vi "LIA Lock-In Simulation.vi"() -> ()   [LabVIEW 2017]
uses:
  <vilib>/Analysis/4window.llb/windowTd.ctl
  <vilib>/measure/maspectr.llb/FFT Power Spectrum and PSD for 1 Chan (CDB).vi
  <instrlib>/niRFSG/niRFSG.llb/niRFSG Fractional Resampling (I-Q).vi
  <vilib>/addons/Digital Filter Design/Multirate.llb/DFD MRate Filtering (Array).vi
  <vilib>/measure/maspectr.llb/FFT Power Spectrum and PSD for 1 Chan.vi
  <vilib>/addons/Digital Filter Design/NI_DigFilterLicensed.lvlib
  <vilib>/ptbypt/NI_PtbyPt.lvlib
  <vilib>/measure/NI_MAPro.lvlib
  <vilib>/Analysis/NI_AALPro.lvlib
panel:
  out "r max - min":dbl=0.5000000090754294 format="%#_6p"
  out "r min":dbl=0.5000000090754294 format="%#_6p"
  out "r max":dbl=0.5000000090754294 format="%#_6p"
  out "Waveform Graph 4":dbl[][](graph) caption="Filtered Response - Time"
  out "r mean":dbl=0.5000000090754294 format="%#_6p"
  in  "sample length":i32=4096
  in  "frequency error (Hz)":dbl format="%#_6p"
  out "Waveform Graph 3":cluster{"f0":dbl, "df":dbl, "magnitude":dbl[]}(graph) caption="Filtered Response - Frequency"
  out "Waveform Graph 2":cluster{"f0":dbl, "df":dbl, "magnitude":dbl[]}[](graph)
  in  "noise":dbl=0.0001 format="%.2p"
  in  "fs":dbl=100000000.0 format="%#_6p"
  in  "decimating factor":i32=1000
  out "error out":errorcluster
  in  "signal freq":dbl=100000.0 format="%#_6p"
  in  "stop":bool
  out "filter response":cluster{"f0":dbl, "df":dbl, "values":dbl[]}[](graph)
  out "Waveform Graph":dbl[][](graph) caption="Filtered Response - Time"
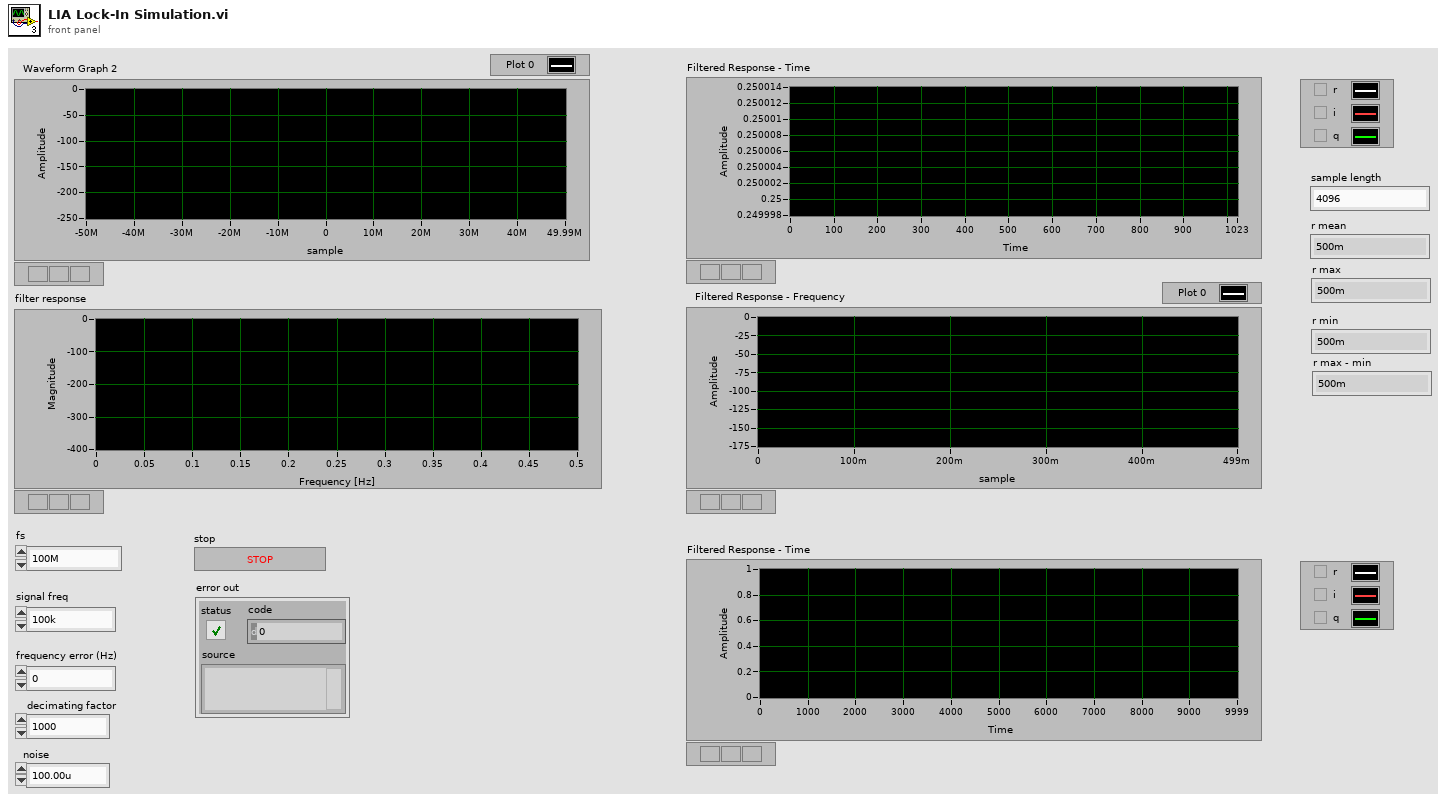
[diagram p1: front panel]
types:
  T1 = typedef "NI_AALPro.lvlib/windowTd.ctl" = u32
  T2 = typedef "NI_DigFilterLicensed.lvlib/DFD Multirate Filter Obj.ctl" = cluster{"mMRate_Structure":enum16{"CIC", "FIR", "IIR", "Lattice"}, "mMRate_Mode":T3, "mMRate_Factor":i32, "mMRate_FIRParams":cluster{"mMRate_FIR_H":dbl[], "mMRate_FIR_IsNyquist?":bool, "mMRate_FIR_IsSymmetric?":bool}, "mMRate_CICParams":cluster{"mMRate_CIC_#Stage":i32, "mMRate_CIC_Lag":i32, "mMRate_CIC_Type":enum16{"Lowpass", "Highpass"}}, "mMRate_Order":i32, "mMRate_Version":string, "mMRate_Comments":string, "mMRate_RationalFactor":cluster{"mMRate_L":i32, "mMRate_M":i32}, "mMRate_Fs":dbl, "mMRate_Quantized?":bool, "mMRate_QFilterGain":dbl, "mMRate_CoefWl":i16, "mMRate_Scaling":cluster{"mMRate_ScaleByPowerOf2?":bool, "mMRate_ScaleType":T4}, "mMRate_InputWl":i16, "mMRate_OutputWl":i16, "mMRate_OutputMode":T5, "mMRate_MultMode":T6, "mMRate_BitPruning":bool, "mMRate_GainWl":i16, "mMRate_OutputFwl":i16, "mMRate_SumIwl":i16, "mMRate_InputIwl ":i16, "mMRate_SumWl":i16, "mMRate_CoefIwl":i16}
  T3 = typedef "NI_DigFilterLicensed.lvlib/DFD Multirate Mode.ctl" = i16
  T4 = typedef "NI_DigFilterLicensed.lvlib/DFD Coef Norm Type.ctl" = enum16{"No Norm", "Time Domain 1-Norm", "Time Domain 2-Norm", "Time Domain Inf-Norm"}
  T5 = typedef "NI_DigFilterLicensed.lvlib/DFD Round-off Mode.ctl" = enum16{"Nearest", "Truncation"}
  T6 = typedef "NI_DigFilterLicensed.lvlib/DFD FXP MRate Multiply Mode.ctl" = enum16{"Truncated", "Full"}
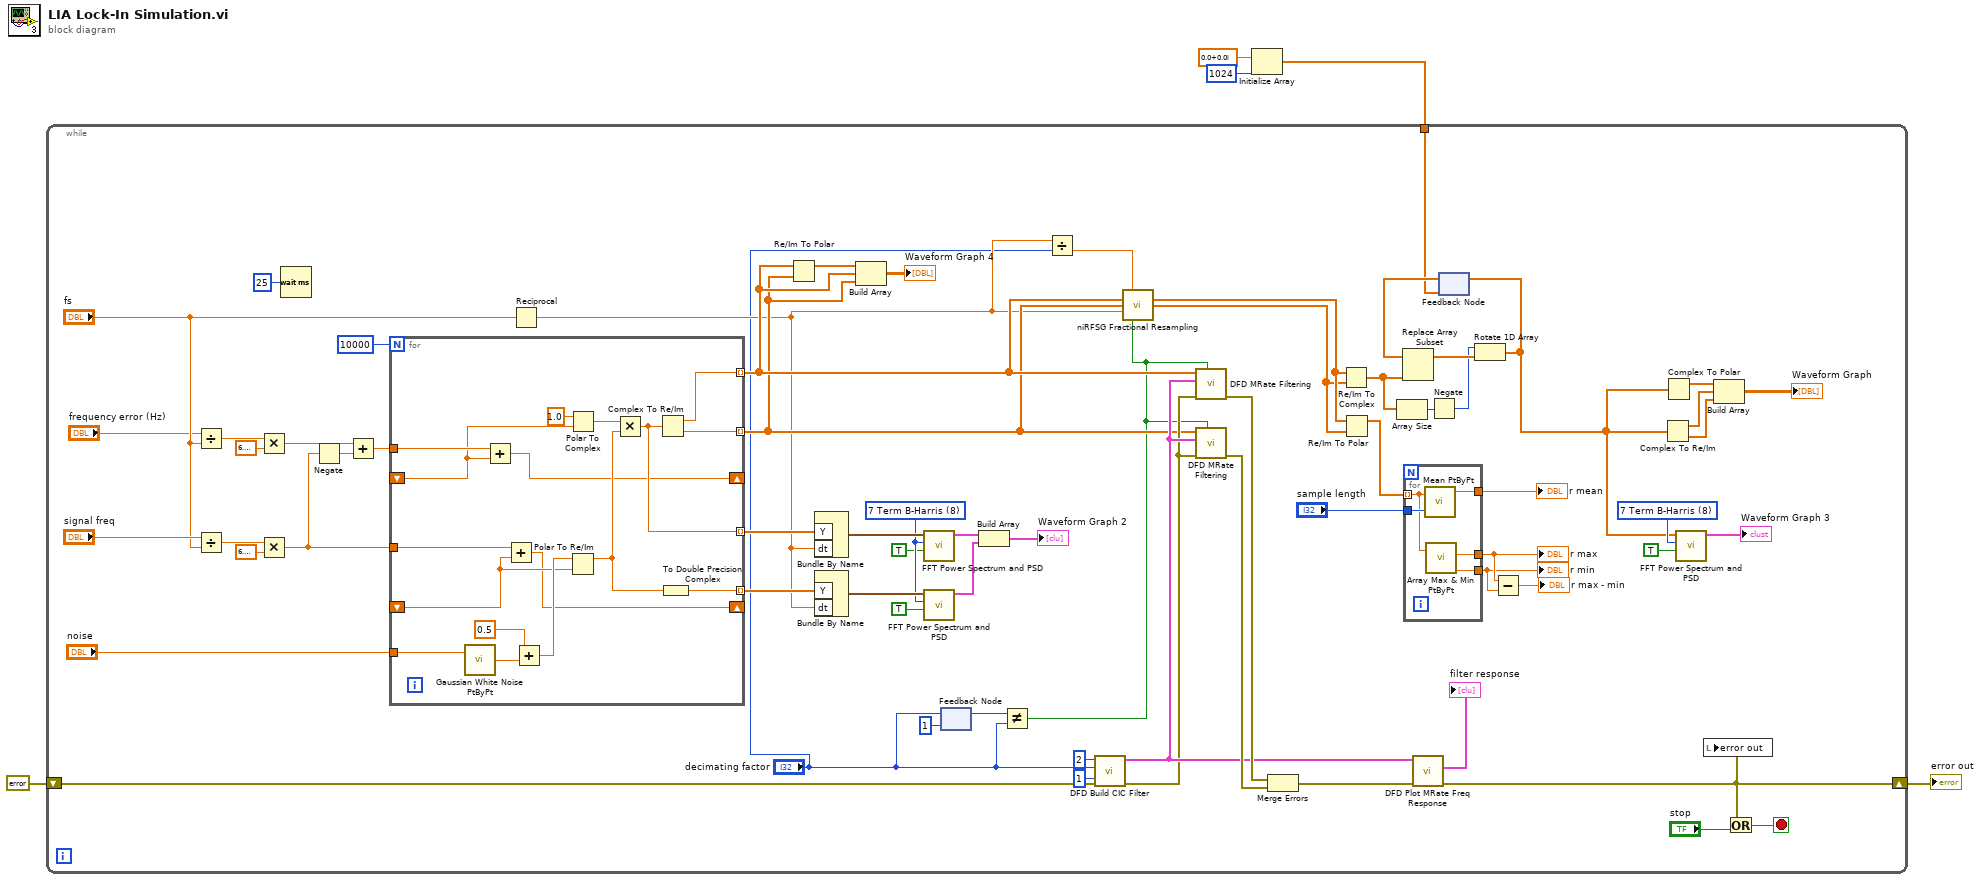
[diagram p0: block diagram]
diagram:
  n1 = Initialize Array(cdb 0.0+0.0i ("element"), 1024 ("dimension size")) -> (w1:cdb[])
  n2 = while {
    shift-right: [w60] -> w5
    shift-left: errorcluster {"status"=FALSE, "code"=0, "source"=""} ("error out") -> [w62]
    tunnel: w1 -> [w26]
    stop <- w67 stop-if-true
    w45 = T1 8 items=["Rectangle"=0, "Hanning"=1, "Hamming"=2, "Blackman-Harris"=3, "Exact Blackman"=4, "Blackman"=5, "Flat Top"=6, "4 Term B-Harris "=7, "7 Term B-Harris"=8, "Low Sidelobe"=9, "Blackman Nuttall"=11, "Triangle"=30, "Bartlett-Hanning"=31, "Bohman"=32, "Parzen"=33, "Welch"=34, "Kaiser"=60, "Dolph-Chebyshev"=61, "Gaussian"=62] ("window")
    w52 = T1 8 items=["Rectangle"=0, "Hanning"=1, "Hamming"=2, "Blackman-Harris"=3, "Exact Blackman"=4, "Blackman"=5, "Flat Top"=6, "4 Term B-Harris "=7, "7 Term B-Harris"=8, "Low Sidelobe"=9, "Blackman Nuttall"=11, "Triangle"=30, "Bartlett-Hanning"=31, "Bohman"=32, "Parzen"=33, "Welch"=34, "Kaiser"=60, "Dolph-Chebyshev"=61, "Gaussian"=62] ("window")
    n3 = Divide(x="frequency error (Hz)", y="fs") -> (x/y=w34:dbl)
    n4 = Divide(x="signal freq", y="fs") -> (x/y=w59:dbl)
    n5 = Multiply(x=w34, y=6.283185307179586) -> (x*y=w30:dbl)
    n6 = Multiply(x=w59, y=6.283185307179586) -> (x*y=w37:dbl)
    n7 = Wait (ms)(milliseconds to wait=u32 25) -> ()  [unwired: 1 out]
    n8 = Negate(x=w37) -> (-x=w41:dbl)
    n9 = Add(x=w30, y=w41) -> (x+y=w36:dbl)
    n10 = for {
      N: 10000 -> [_]
      tunnel: w36 -> [w83]
      tunnel: [w93] -> w13 mode=indexing
      tunnel: [w92] -> w12 mode=indexing
      tunnel: w37 -> [w82]
      tunnel: "noise" -> [w88]
      tunnel: [w85] -> w55 mode=indexing
      tunnel: [w86] -> w56 mode=indexing
      shift-right: [w84] -> _
      shift-left: _ -> [w79]
      shift-right: [w80] -> _
      shift-left: _ -> [w81]
      n11 = call <vilib>:"Gaussian White Noise PtByPt.vi"("standard deviation"=w88) -> ("Gaussian white noise"=w91:dbl)  [unwired: 2 in]
      n12 = Add(x=w83, y=w79) -> (x+y=w84:dbl)
      n13 = Add(x=w82, y=w81) -> (x+y=w80:dbl)
      n14 = Add(x=0.5 ("r"), y=w91) -> (x+y=w89:dbl)
      n15 = Polar To Complex(1:w79, 2:1.0 ("r")) -> (0:w94:cdb)
      n16 = Polar To Re/Im(2:w81, 3:w89) -> (1:w87:dbl)  [unwired: 1 out]
      n17 = Multiply(x=w94, y=w87) -> (x*y=w86:cdb)
      n18 = Complex To Re/Im(x + iy=w86) -> (x=w93:dbl, y=w92:dbl)
      n19 = To Double Precision Complex(1:w87) -> (0:w85:cdb)
    }
    n20 = Reciprocal(x="fs") -> (1/x=w11:dbl)
    n21 = Re/Im To Polar(2:w12, 3:w13) -> (1:w19:dbl[])  [unwired: 1 out]
    n22 = Bundle By Name("Y"=w56, "dt"=w11) -> (w54:waveform(cdb))  [unwired: 1 in]
    n23 = Bundle By Name("Y"=w55, "dt"=w11) -> (w53:waveform(cdb))  [unwired: 1 in]
    n24 = Build Array(w19, w13, w12) -> (→"Waveform Graph 4":dbl[][])
    n25 = call-poly <vilib>:"FFT Power Spectrum and PSD.vi"("dB On (F)"=TRUE, "window"=w52, "time signal"=w54) -> ("Power Spectrum / PSD"=w49:cluster{"f0":dbl, "df":dbl, "magnitude":dbl[]})  [unwired: 5 in, 3 out]
    n26 = call-poly <vilib>:"FFT Power Spectrum and PSD.vi"("dB On (F)"=TRUE, "window"=w52, "time signal"=w53) -> ("Power Spectrum / PSD"=w48:cluster{"f0":dbl, "df":dbl, "magnitude":dbl[]})  [unwired: 5 in, 3 out]
    n27 = feedback-in #1("decimating factor") -> ()
    n28 = feedback #1(1 ("decimating factor")) -> (w43:i32)
    n29 = Build Array(w49, w48) -> (→"Waveform Graph 2":cluster{"f0":dbl, "df":dbl, "magnitude":dbl[]}[])
    n30 = Not Equal?(x=w43, y="decimating factor") -> (x != y?=w8:bool)
    n31 = Divide(x=w11, y="decimating factor") -> (x/y=w10:dbl)
    n32 = call <vilib>:"DFD Build CIC Filter.vi"("error in (no error)"=w62, "differential delay"=1, "factor"="decimating factor", "# stages"=2) -> ("error out"=w61:errorcluster, "CIC filter out"=w63:T2)  [unwired: 6 in]
    n33 = call-poly <instrlib>:"niRFSG Fractional Resampling.vi"("desired sample rate (Hz)"=w10, "I"=w13, "Q"=w12, "input sample rate"=w11, "reset? (T)"=w8) -> ("I out"=w7:dbl[], "Q out"=w6:dbl[])  [unwired: 8 in, 1 out]
    n34 = call-poly <vilib>:"DFD MRate Filtering.vi"("init? (F)"=w8, "error in (no error)"=w61, "multirate filter"=w63, "signal in"=w13) -> ("error out"=w65:errorcluster)  [unwired: 6 in, 1 out]
    n35 = call-poly <vilib>:"DFD MRate Filtering.vi"("init? (F)"=w8, "error in (no error)"=w61, "multirate filter"=w63, "signal in"=w12) -> ("error out"=w68:errorcluster)  [unwired: 6 in, 1 out]
    n36 = Merge Errors(w65, w68) -> (w66:errorcluster)
    n37 = Re/Im To Complex(1:w6, 2:w7) -> (0:w28:cdb[])
    n38 = Re/Im To Polar(2:w6, 3:w7) -> (1:w24:dbl[])  [unwired: 1 out]
    n39 = Array Size(array=w28) -> (size(s)=w25:i32)
    n40 = for {
      tunnel: w24 -> [w76] mode=indexing
      tunnel: "sample length" -> [w78]
      tunnel: [w77] -> w22
      tunnel: [w75] -> w16
      tunnel: [w74] -> w15
      n41 = call <vilib>:"Mean PtByPt.vi"("x"=w76, "sample length"=w78) -> ("mean"=w77:dbl)  [unwired: 2 in, 1 out]
      n42 = call <vilib>:"Array Max & Min PtByPt.vi"("input data point"=w76) -> ("max value"=w75:dbl, "min value"=w74:dbl)  [unwired: 2 in, 3 out]
    }
    "r mean" <- w22
    "r max" <- w16
    "r min" <- w15
    n43 = call <vilib>:"DFD Plot MRate Freq Response.vi"("error in (no error)"=w66, "multirate filter in"=w63) -> ("error out"=w60:errorcluster, "magnitude response"=→"filter response":cluster{"f0":dbl, "df":dbl, "values":dbl[]}[])  [unwired: 6 in, 2 out]
    n44 = Negate(x=w25) -> (-x=w17:i32)
    n45 = feedback #2(w26) -> (w27:cdb[])
    n46 = Replace Array Subset(array=w27, new element=w28) -> (w29:cdb[])  [unwired: 1 in]
    n47 = Rotate 1D Array(1:w29, 2:w17) -> (0:w18:cdb[])
    n48 = feedback-in #2(w18) -> ()
    n49 = Subtract(x=w16, y=w15) -> (x-y=→"r max - min":dbl)
    n50 = Complex To Re/Im(x + iy=w18) -> (x=w40:dbl[], y=w38:dbl[])
    n51 = Complex To Polar(r * e^(i*theta)=w18) -> (r=w35:dbl[])  [unwired: 1 out]
    n52 = call-poly <vilib>:"FFT Power Spectrum and PSD.vi"("dB On (F)"=TRUE, "window"=w45, "time signal"=w18) -> ("Power Spectrum / PSD"=→"Waveform Graph 3":cluster{"f0":dbl, "df":dbl, "magnitude":dbl[]})  [unwired: 5 in, 3 out]
    n53 = local write "error out"(w60) -> ()
    n54 = Build Array(w35, w40, w38) -> (→"Waveform Graph":dbl[][])
    n55 = Or(x=w60, y="stop") -> (x .or. y?=w67:bool)
  }
  "error out" <- w5
